vi "pipette_to_cam.vi"(7 "which manipulator":T2(ring), 9 "transform cluster + actuator":T3, 10 "current positions":T1, 11 "pipette position (steps)":i32[](array[numeric])) -> (3 "pipette position (px)":dbl[](array[numeric]))   [LabVIEW 2015]
uses:
  pipette cleaning/pressure box/cleaning_soft/controls/actuator_type.ctl
  pipette cleaning/pressure box/cleaning_soft/controls/actuator_cluster.ctl
  transform_properties_actuators.ctl
  controls/transform_cluster_actuator.ctl
panel:
  # "pipette (steps) to cam (px)"
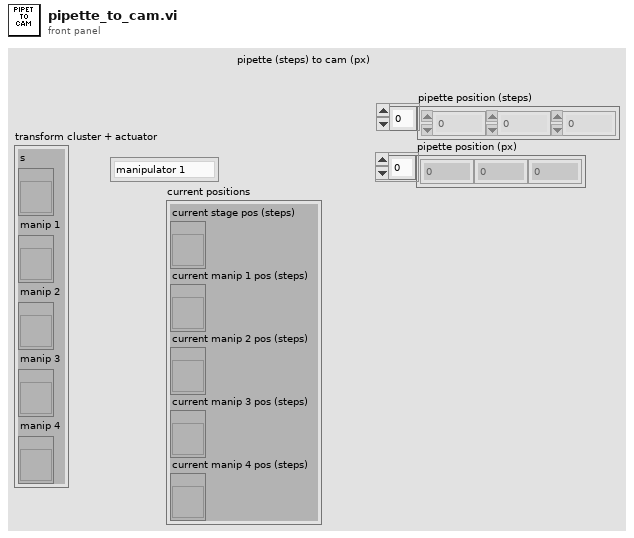
[diagram p1: front panel]
types:
  T1 = cluster{"current stage pos (steps)":refnum<vi>, "current manip 1 pos (steps)":refnum<vi>, "current manip 2 pos (steps)":refnum<vi>, "current manip 3 pos (steps)":refnum<vi>, "current manip 4 pos (steps)":refnum<vi>}
  T2 = enum16{"manipulator 1", "manipulator 2", "manipulator 3", "manipulator 4"}
  T3 = typedef "transform_cluster_actuator.ctl" = cluster{"s":refnum<vi>, "manip 1":refnum<vi>, "manip 2":refnum<vi>, "manip 3":refnum<vi>, "manip 4":refnum<vi>}
  T4 = typedef "transform_properties_actuators.ctl" = cluster{"theta (deg)":dbl, "X sc factor (px/step)":dbl, "Y sc factor (px/step)":dbl, "zero loc (x,y,z)":dbl[], "flip y?":bool, "flip x?":bool, "gamma (deg)":dbl, "flip z?":bool, "Z sc factor (px/step)":dbl, "actuator":T5, "safe space (steps)":i32[]}
  T5 = typedef "actuator_cluster.ctl" = cluster{"Actuator COM":refnum<visa-resource-name>, "Actuator type":T6}
  T6 = typedef "actuator_type.ctl" = enum16{"Scientifica", "Sutter", "Demo", "Off"}
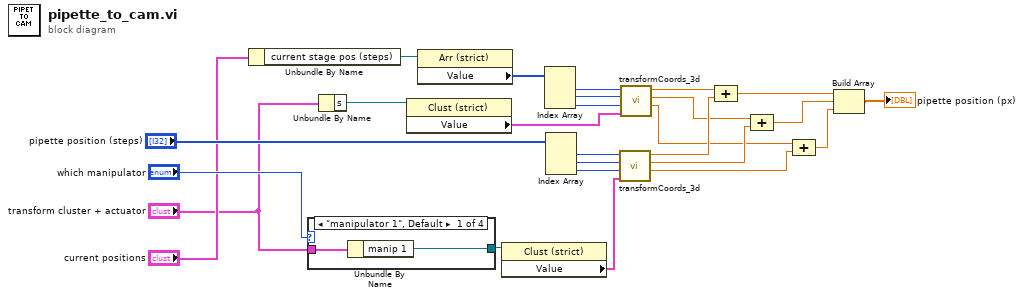
[diagram p0: block diagram]
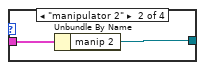
[diagram p2: hidden frame]
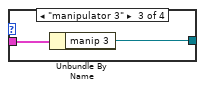
[diagram p3: hidden frame]
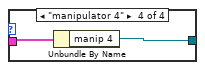
[diagram p4: hidden frame]
diagram:
  n1 = Unbundle By Name("current positions") -> ("current stage pos (steps)"=w18:refnum<vi>)
  n2 = case shown="\"manipulator 1\", Default" "which manipulator" {
    tunnel: "transform cluster + actuator" -> [w28 w30 w32 w34]
    tunnel: [w27 w29 w31 w33] -> w21
    frame "manipulator 1", Default {
      n3 = Unbundle By Name(w28) -> ("manip 1"=w27:refnum<vi>)
    }
    frame "manipulator 2" {
      n4 = Unbundle By Name(w30) -> ("manip 2"=w29:refnum<vi>)
    }
    frame "manipulator 3" {
      n5 = Unbundle By Name(w32) -> ("manip 3"=w31:refnum<vi>)
    }
    frame "manipulator 4" {
      n6 = Unbundle By Name(w34) -> ("manip 4"=w33:refnum<vi>)
    }
  }
  n7 = Unbundle By Name("transform cluster + actuator") -> ("s"=w12:refnum<vi>)
  n8 = property class="Clust (strict)"(reference=w12) -> ("Value"=w11:T4)  [unwired: 1 in, 2 out]
  n9 = property class="Arr (strict)"(reference=w18) -> ("Value"=w17:i32[])  [unwired: 1 in, 2 out]
  n10 = property class="Clust (strict)"(reference=w21) -> ("Value"=w20:T4)  [unwired: 1 in, 2 out]
  n11 = Index Array(array=w17) -> (element #1=w16:i32, element #2=w15:i32, element #3=w14:i32)  [unwired: 3 in]
  n12 = Index Array(array="pipette position (steps)") -> (element #1=w26:i32, element #2=w25:i32, element #3=w24:i32)  [unwired: 3 in]
  n13 = call "transformCoords_3d.vi"("transform properties"=w20, "z"=w24, "y"=w25, "x"=w26) -> ("z out"=w5:dbl, "y out"=w7:dbl, "x out"=w9:dbl)  [unwired: 5 in]
  n14 = call "transformCoords_3d.vi"("transform properties"=w11, "z"=w14, "y"=w15, "x"=w16) -> ("z out"=w6:dbl, "y out"=w8:dbl, "x out"=w10:dbl)  [unwired: 5 in]
  n15 = Compound Arithmetic op=ADD(w10, w9) -> (w4:dbl)
  n16 = Compound Arithmetic op=ADD(w8, w7) -> (w3:dbl)
  n17 = Compound Arithmetic op=ADD(w6, w5) -> (w2:dbl)
  n18 = Build Array(w4, w3, w2) -> (→"pipette position (px)":dbl[])
